vi "Add New Or Old Label.vi"(8 "old label?":bool, 9 "refresh listbox":T7[](array[typedef]), 10 "label":T1) -> (1 "refresh listbox out":T7[](array[typedef]))   [LabVIEW 2020, in "Ballard ARINC 429 System Explorer.lvlib" / "Implementation.lvlib"]
uses:
  Implementation.lvlib
  Types/Refresh Listbox.ctl
  Types/Refresh Symbols.ctl
  Shared/VS Channels Definition for Label.ctl
  Shared/VS Channel Definition for Parameter.ctl
  Shared/Direction.ctl
  Shared/Parameter Definition.ctl
  Encoding and Decoding/Encoding.ctl
  Shared/Transfer Type.ctl
  Refresh Constants.vi
  Encoding and Decoding/Encoding and Decoding.lvlib
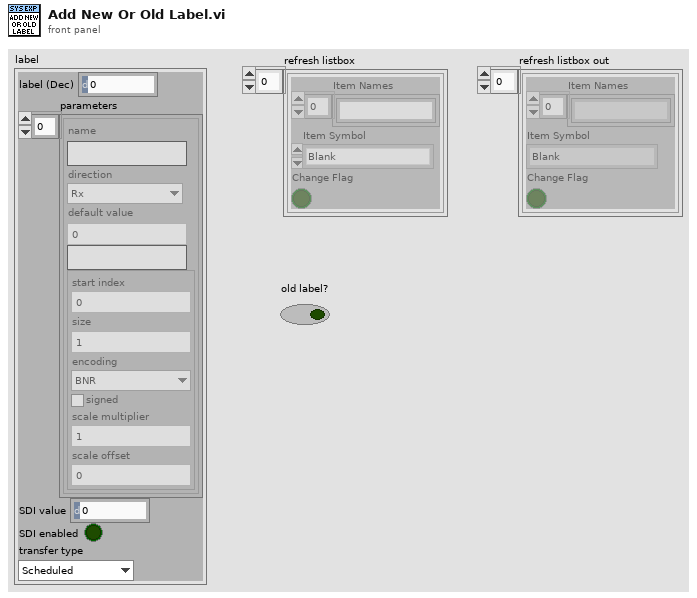
[diagram p1: front panel]
types:
  T1 = typedef "VS Channels Definition for Label.ctl" = cluster{"label (Dec)":u32, "parameters":T2[], "SDI value":u8, "SDI enabled":bool, "transfer type":T6}
  T2 = typedef "VS Channel Definition for Parameter.ctl" = cluster{"name":string, "direction":T3, "default value":dbl, "unit":string, "Parameter":T4}
  T3 = typedef "Direction.ctl" = enum16{"Rx", "Tx"}
  T4 = typedef "Parameter Definition.ctl" = cluster{"start index":i32, "size":i32, "encoding":T5, "signed":bool, "scale multiplier":dbl, "scale offset":dbl}
  T5 = typedef "Encoding and Decoding.lvlib/Encoding.ctl" = enum16{"BNR", "BCD", "Discrete"}
  T6 = typedef "Transfer Type.ctl" = enum16{"Scheduled", "Acyclic", "Block", "Strobe"}
  T7 = typedef "Ballard ARINC 429 System Explorer.lvlib/Implementation.lvlib/Refresh Listbox.ctl" = cluster{"Item Names":string[], "Item Symbol":T8, "Change Flag":bool}
  T8 = typedef "Ballard ARINC 429 System Explorer.lvlib/Implementation.lvlib/Refresh Symbols.ctl" = enum16{"Blank", "Port", "Incoming", "Outgoing", "Label", "Word", "Parameter", "ARINC-429", "Config Files", "Channel Spec", "Item"}
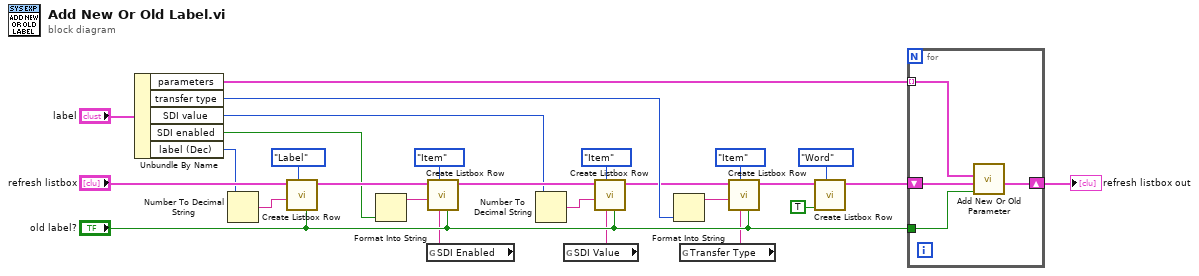
[diagram p0: block diagram]
diagram:
  n1 = Unbundle By Name("label") -> ("parameters"=w11:T2[], "transfer type"=w13:T6, "SDI value"=w17:u8, "SDI enabled"=w2:bool, "label (Dec)"=w22:u32)
  n2 = Number To Decimal String(number=w22) -> (decimal integer string=w24:string)  [unwired: 1 in]
  n3 = call "Create Listbox Row.vi"("swap new and old (F)"="old label?", "refresh symbol (Blank)"=Refresh_Symbols."Label" ("Refresh Symbol (Blank)"), "new item"=w24, "refresh listbox"="refresh listbox") -> ("refresh listbox out"=w20:T7[])  [unwired: 7 in]
  n4 = Format Into String(w2) -> (resulting string=w1:string)  [unwired: 3 in, 1 out]
  n5 = global read "Refresh Constants.vi" "SDI Enabled"() -> (w5:string)
  n6 = call "Create Listbox Row.vi"("swap new and old (F)"="old label?", "override name"=w5, "refresh symbol (Blank)"=Refresh_Symbols."Item" ("Refresh Symbol (Blank)"), "new item"=w1, "refresh listbox"=w20) -> ("refresh listbox out"=w18:T7[])  [unwired: 6 in]
  n7 = Number To Decimal String(number=w17) -> (decimal integer string=w19:string)  [unwired: 1 in]
  n8 = global read "Refresh Constants.vi" "SDI Value"() -> (w4:string)
  n9 = call "Create Listbox Row.vi"("swap new and old (F)"="old label?", "override name"=w4, "refresh symbol (Blank)"=Refresh_Symbols."Item" ("Refresh Symbol (Blank)"), "new item"=w19, "refresh listbox"=w18) -> ("refresh listbox out"=w12:T7[])  [unwired: 6 in]
  n10 = Format Into String(w13) -> (resulting string=w14:string)  [unwired: 3 in, 1 out]
  n11 = global read "Refresh Constants.vi" "Transfer Type"() -> (w3:string)
  n12 = call "Create Listbox Row.vi"("swap new and old (F)"="old label?", "override name"=w3, "refresh symbol (Blank)"=Refresh_Symbols."Item" ("Refresh Symbol (Blank)"), "new item"=w14, "refresh listbox"=w12) -> ("refresh listbox out"=w9:T7[])  [unwired: 6 in]
  n13 = call "Create Listbox Row.vi"("refresh symbol (Blank)"=Refresh_Symbols."Word" ("Refresh Symbol (Blank)"), "change? (T)"=TRUE, "refresh listbox"=w9) -> ("refresh listbox out"=w8:T7[])  [unwired: 8 in]
  n14 = for {
    shift-right: [w28] -> w25
    shift-left: w8 -> [w31]
    tunnel: w11 -> [w29] mode=indexing
    tunnel: "old label?" -> [w30]
    n15 = call "Add New Or Old Parameter.vi"("old port?"=w30, "refresh listbox"=w31, "channel parameter"=w29) -> ("refresh listbox out"=w28:T7[])  [unwired: 8 in]
  }
  "refresh listbox out" <- w25
